vi "rad_Extract Full Image.vi"(6 "Subfolder (lvappimage.contents)":string="lvappimage.contents", 8 "error in (no error)":errorcluster, 10 "App Image Temp Folder":path, 11 "Zipped App Image File Path":path) -> (0 "error out":errorcluster, 3 "Unzipped App Image Folder Path":path)   [LabVIEW 2020]
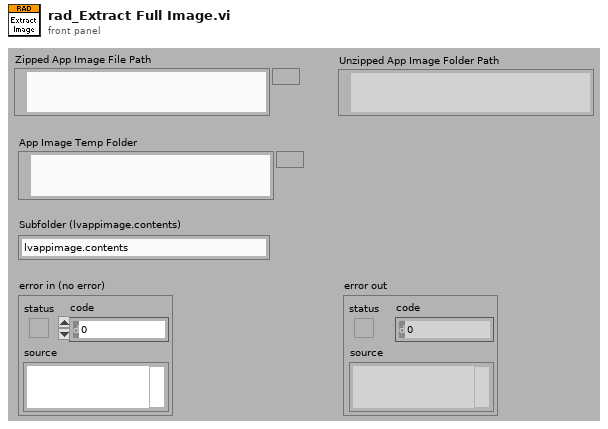
[diagram p1: front panel]
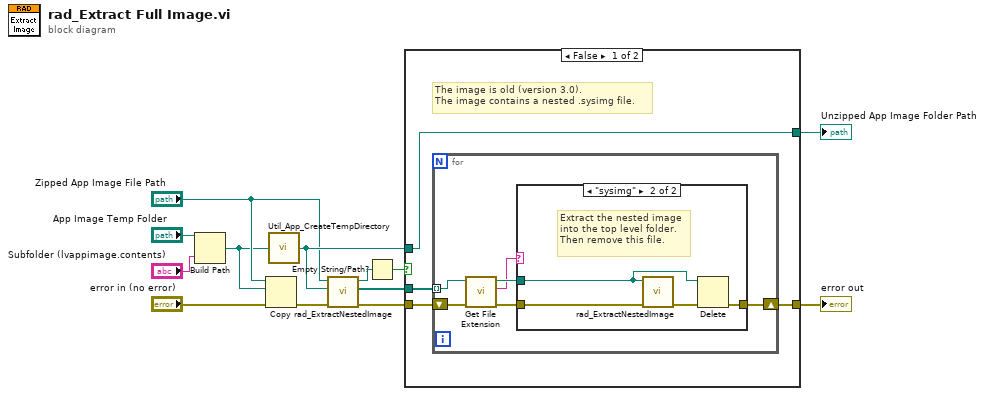
[diagram p0: block diagram]
diagram:
  n1 = Build Path(base path="App Image Temp Folder", name or relative path="Subfolder (lvappimage.contents)") -> (appended path=w2:path)
  n2 = Copy(8:"error in (no error)", 10:w2, 11:"Zipped App Image File Path") -> (0:w4:errorcluster)  [unwired: 2 in, 2 out]
  n3 = call "Util_App_CreateTempDirectory.vi"("TempFolderPath"=w2) -> ("TempFolderPath_out"=w8:path)
  n4 = call "rad_ExtractNestedImage.vi"("error in"=w4, "TempFolderPath"=w8, "image file path"="Zipped App Image File Path") -> ("error out"=w11:errorcluster, "Unzipped files"=w9:path[], "NestedImagePath"=w13:path)  [unwired: 6 in]
  n5 = Empty String/Path?(string/path=w13) -> (empty?=w12:bool)
  n6 = case shown="False" w12 {
    tunnel: w11 -> [w16 w30]
    tunnel: [w15 w30] -> w10
    tunnel: w9 -> [w17 _]
    tunnel: w8 -> [w14 w29]
    tunnel: [w14 w29] -> w7
    frame False {
      # "The image is old (version 3.0).\nThe image contains a nested .sysimg file."
      n7 = for {
        tunnel: w17 -> [w20] mode=indexing
        shift-right: [w23] -> w15
        shift-left: w16 -> [w22]
        n8 = call <vilib>:"Get File Extension.vi"("error in (no error)"=w22, "file"=w20) -> ("error out"=w21:errorcluster, "lowercase file extension"=w18:string, "dup file"=w19:path)  [unwired: 5 in, 2 out]
        n9 = case shown="\"sysimg\"" w18 {
          tunnel: w21 -> [w24 w28]
          tunnel: w19 -> [_ w27]
          tunnel: [w24 w25] -> w23
          frame Default {
            # "Leave other files alone\nin the top level folder."
          }
          frame "sysimg" {
            # "Extract the nested image\ninto the top level folder.\nThen remove this file."
            n10 = call "rad_ExtractNestedImage.vi"("error in"=w28, "image file path"=w27) -> ("error out"=w26:errorcluster)  [unwired: 7 in, 2 out]
            n11 = Delete(path (use dialog)=w27, error in=w26) -> (error out=w25:errorcluster)  [unwired: 3 in, 2 out]
          }
        }
      }
    }
    frame True {
      # "This image is new (version 5.5).\nThe contents are compressed once."
    }
  }
  "Unzipped App Image Folder Path" <- w7
  "error out" <- w10
